vi "ElevatorSim_New.vi"(4 "Simulate Gravity":bool=TRUE, 5 "MaxHeight_Meters":dbl, 6 "DrumRadius_Meters":dbl, 7 "MinHeight_Meters":dbl, 8 "MeasurementStdDev":T1=[[0.0]], 9 "CarriageMass_Kg":dbl, 10 "Gearing":dbl=1.0, 11 "GearBox":T2 {"Jr_KgM2" format="%13.5p"; "L_H" format="%13.5p"; "Kt_NMPerAmp" format="%13.5p"; "KvINV_RadPerSecPerVolt" format="%13.5p"; "R_Ohms" format="%13.5p"; "FreeSpeed_RadPerSec" format="%13.5p"; "FreeCurrent_Amps" format="%13.5p"; "StallCurrent_Amps" format="%13.5p"; "StallTorque_NM" format="%13.5p"; "nominalVoltage_Volts" format="%13.5p"}) -> (0 "Error":bool, 3 "ElevatorSim":T3={"LinearSystemSim"={"m_Plant"={"m_A"=[], "m_B"=[], "m_C"=[], "m_D"=[], "States"=0, "Inputs"=0, "Outputs"=0}, "m_X"=[], "m_Y"=[], "m_U"=[], "MeasureStdDev"=[]}, "GearBox"={"nominalVoltage_Volts"=0.0, "StallTorque_NM"=0.0, "StallCurrent_Amps"=0.0, "FreeCurrent_Amps"=0.0, "FreeSpeed_RadPerSec"=0.0, "R_Ohms"=0.0, "KvINV_RadPerSecPerVolt"=0.0, "Kt_NMPerAmp"=0.0, "L_H"=0.0, "Jr_KgM2"=0.0}, "Gearing"=0.0, "DrumRadius_M"=0.0, "MinHeight_M"=0.0, "MaxHeight_M"=0.0, "CarriageMass_Kg"=0.0, "SimulateGravity"=TRUE} {"GearBox"."Jr_KgM2" format="%13.5p"; "GearBox"."L_H" format="%13.5p"; "GearBox"."Kt_NMPerAmp" format="%13.5p"; "GearBox"."KvINV_RadPerSecPerVolt" format="%13.5p"; "GearBox"."R_Ohms" format="%13.5p"; "GearBox"."FreeSpeed_RadPerSec" format="%13.5p"; "GearBox"."FreeCurrent_Amps" format="%13.5p"; "GearBox"."StallCurrent_Amps" format="%13.5p"; "GearBox"."StallTorque_NM" format="%13.5p"; "GearBox"."nominalVoltage_Volts" format="%13.5p"})   [LabVIEW 2019, in "Trajectory_Library.lvlib"]
doc: "Creates a simulated elevator mechanism.\n \nInputs:\n - maxHeightMeters -- The max allowable height of the elevator.\n - minHeightMeters -- The min allowable height of the elevator.\n - gearbox -- The type of and number of motors in the elevator gearbox.\n - gearing -- The gearing of the elevator (numbers greater than 1 represent reductions).\n - carriageMassKg -- The mass of the elevator carriage.\n - MeasurementStdDev -- Vector matrix of std deviations for measurements.\n - drumRadiusMeters -- The radius of the drum that the elevator spool is wrapped around.\n - SimulateGravity -- Simulate gravity (optional) Default: True\n\nOutputs:\n - OutElevatorSim -- Updated data cluster\n - Error -- If TRUE, an error occured."
uses:
  Trajectory_Library.lvlib
  <vilib>/Analysis/Matrix/Datatypes/RealMatrix.ctl
  <vilib>/Analysis/Matrix/NI_Matrix.lvlib
  TypeDef/LINEAR_SYSTEM.ctl
  TypeDef/DCMOTOR.CTL
  TypeDef/LINEAR_SYSTEM_SIM.ctl
  TypeDef/ELEVATOR_SIM.ctl
panel:
  # "<1, 1>"
  # "<States, 1>"
  # "<Outputs, 1>"
  # "<Inputs, 1>"
  # "<Outputs, 1>"
  # "<States,States>"
  # "<States,Inputs>"
  # "<Outputs,States>"
  # "<Outputs,Inputs>"
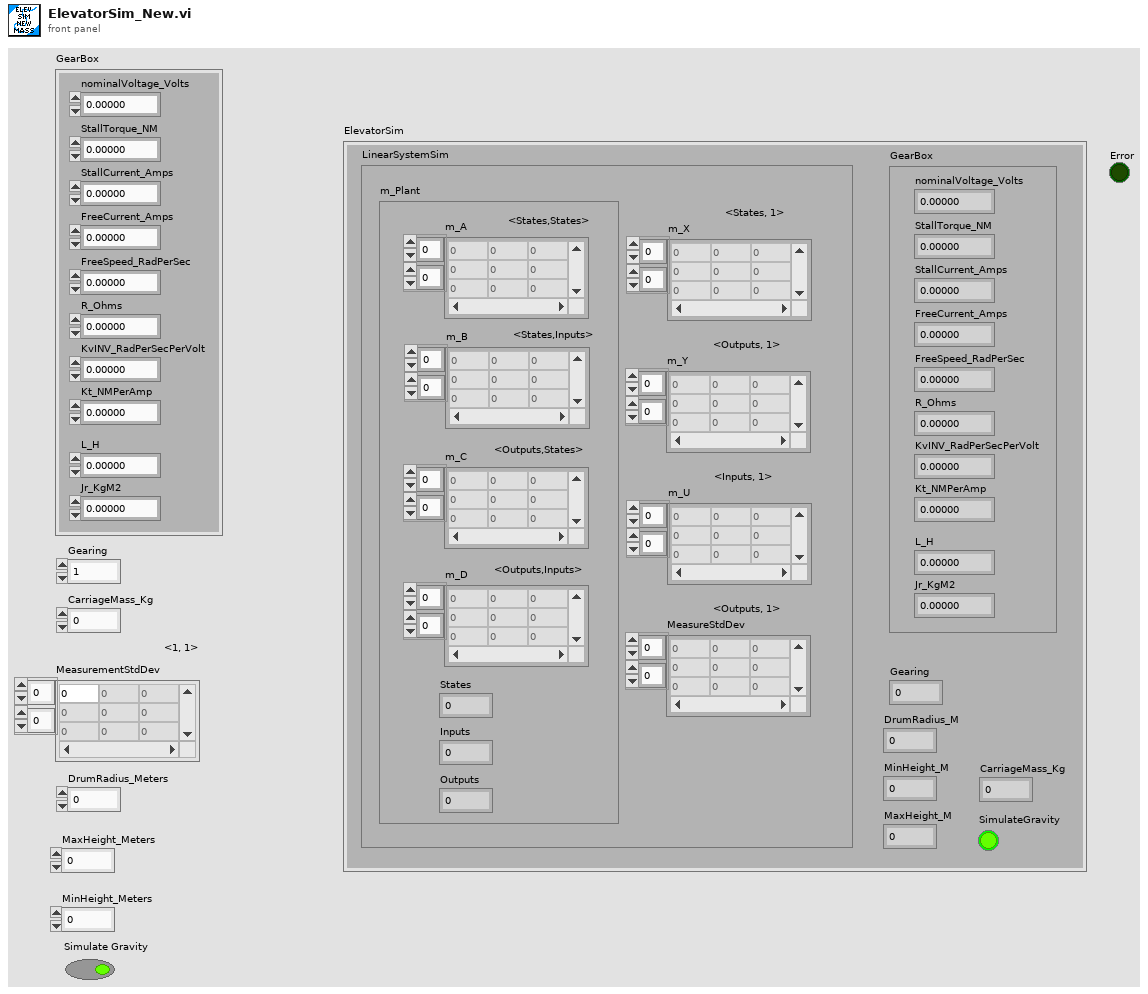
[diagram p1: front panel]
types:
  T1 = typedef "NI_Matrix.lvlib/RealMatrix.ctl" = dbl[][]
  T2 = typedef "Trajectory_Library.lvlib/DCMOTOR.CTL" = cluster{"nominalVoltage_Volts":dbl, "StallTorque_NM":dbl, "StallCurrent_Amps":dbl, "FreeCurrent_Amps":dbl, "FreeSpeed_RadPerSec":dbl, "R_Ohms":dbl, "KvINV_RadPerSecPerVolt":dbl, "Kt_NMPerAmp":dbl, "L_H":dbl, "Jr_KgM2":dbl}
  T3 = typedef "Trajectory_Library.lvlib/ELEVATOR_SIM.ctl" = cluster{"LinearSystemSim":T4, "GearBox":T2, "Gearing":dbl, "DrumRadius_M":dbl, "MinHeight_M":dbl, "MaxHeight_M":dbl, "CarriageMass_Kg":dbl, "SimulateGravity":bool}
  T4 = typedef "Trajectory_Library.lvlib/LINEAR_SYSTEM_SIM.ctl" = cluster{"m_Plant":T5, "m_X":T1, "m_Y":T1, "m_U":T1, "MeasureStdDev":T1}
  T5 = typedef "Trajectory_Library.lvlib/LINEAR_SYSTEM.ctl" = cluster{"m_A":T1, "m_B":T1, "m_C":T1, "m_D":T1, "States":i32, "Inputs":i32, "Outputs":i32}
  T6 = typedef "WPILib_Math.lvlib/LINEAR_SYSTEM.ctl" = cluster{"m_A":T1, "m_B":T1, "m_C":T1, "m_D":T1, "States":i32, "Inputs":i32, "Outputs":i32}
  T7 = typedef "WPILib_Math.lvlib/LINEAR_SYSTEM_SIM.ctl" = cluster{"m_Plant":T6, "m_X":T1, "m_Y":T1, "m_U":T1, "MeasureStdDev":T1}
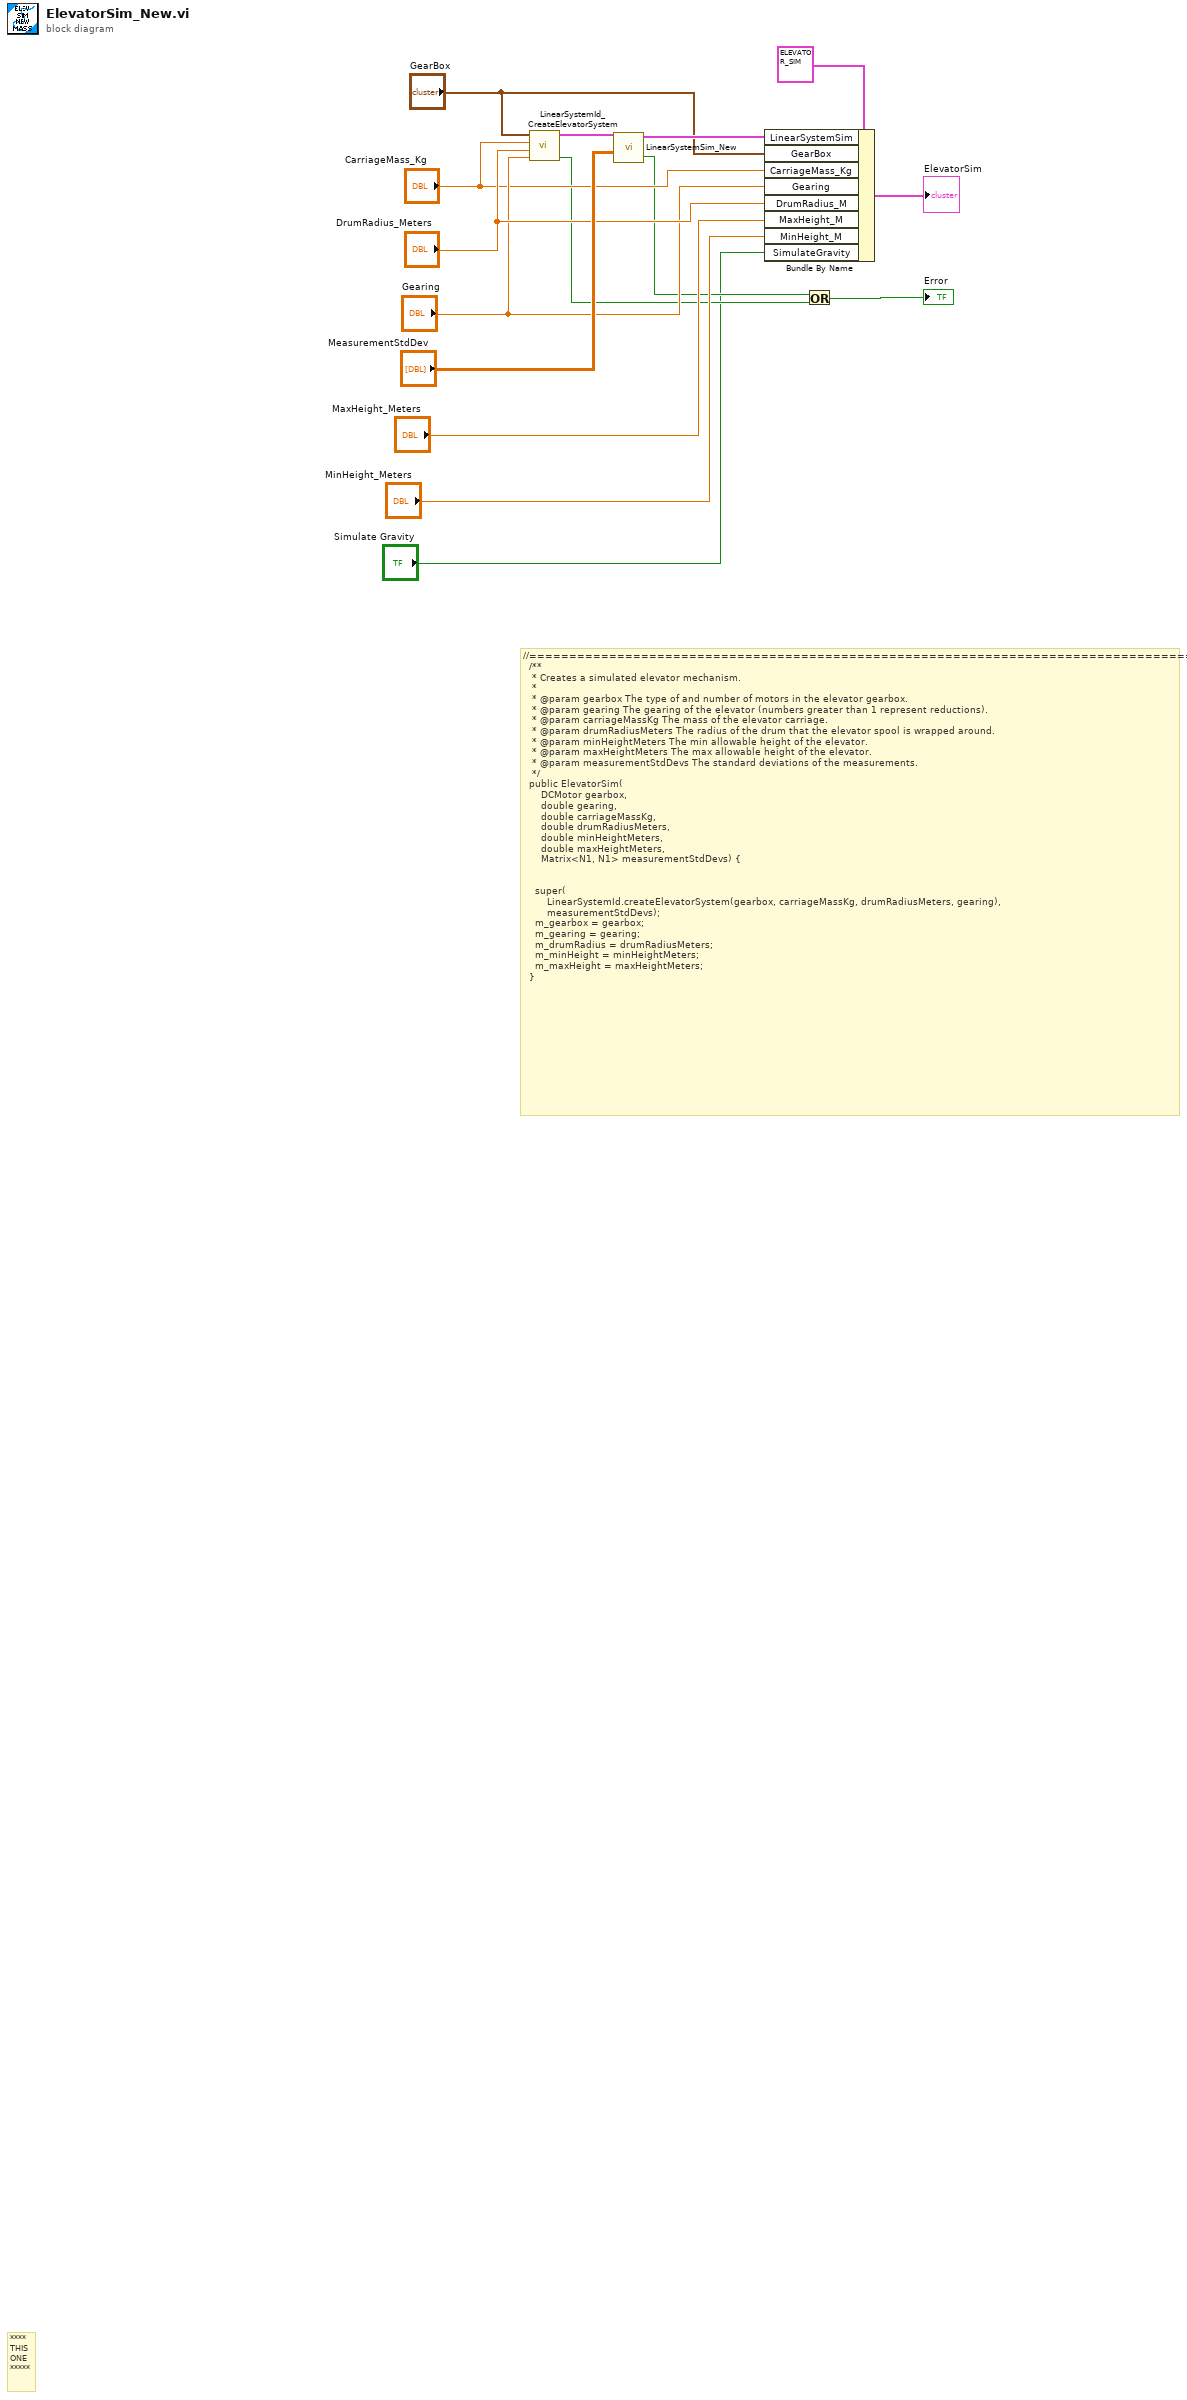
[diagram p0: block diagram]
diagram:
  # "//===================================================================================\n  /**\n   * Creates a simulated elevator mechanism.\n   *\n   * @param gearbox The type of and number of motors in the elevator gearbox.\n   * @param gearing The gearing of the elevator (numbers greater than 1 represent reductions).\n   * @param carriageMassKg The mass of the elevator carriage.\n   * @param drumRadiusMeters The radius of the drum that the elevator spool is wrapped around.\n   * @param minHeightMeters The min allowable height of the elevator.\n   * @param maxHeightMeters The max allowable height of the elevator.\n   * @param measurementStdDevs The standard deviations of the measurements.\n   */\n  public ElevatorSim(\n      DCMotor gearbox,\n      double gearing,\n      double carriageMassKg,\n      double drumRadiusMeters,\n      double minHeightMeters,\n      double maxHeightMeters,\n      Matrix<N1, N1> measurementStdDevs) {\n\n\n    super(\n        LinearSystemId.createElevatorSystem(gearbox, carriageMassKg, drumRadiusMeters, gearing),\n        measurementStdDevs);\n    m_gearbox = gearbox;\n    m_gearing = gearing;\n    m_drumRadius = drumRadiusMeters;\n    m_minHeight = minHeightMeters;\n    m_maxHeight = maxHeightMeters;\n  }"
  # "****\nTHIS\nONE\n*****"
  n1 = call "LinearSystemId_CreateElevatorSystem.vi"("G"="Gearing", "radiusMeters"="DrumRadius_Meters", "massKg"="CarriageMass_Kg", "DCMOTOR"="GearBox") -> ("Size Coerced"=w3:bool, "Linearsystem"=w11:T6)  [unwired: 6 in]
  n2 = call "LinearSystemSim_New.vi"("MeasurementStdDev"="MeasurementStdDev", "System"=w11) -> ("Size Coerced"=w4:bool, "LinearSystemSim"=w13:T7)  [unwired: 8 in]
  n3 = Bundle By Name(cluster=T3 {"LinearSystemSim"={"m_Plant"={"m_A"=[], "m_B"=[], "m_C"=[], "m_D"=[], "States"=0, "Inputs"=0, "Outputs"=0}, "m_X"=[], "m_Y"=[], "m_U"=[], "MeasureStdDev"=[]}, "GearBox"={"nominalVoltage_Volts"=0.0, "StallTorque_NM"=0.0, "StallCurrent_Amps"=0.0, "FreeCurrent_Amps"=0.0, "FreeSpeed_RadPerSec"=0.0, "R_Ohms"=0.0, "KvINV_RadPerSecPerVolt"=0.0, "Kt_NMPerAmp"=0.0, "L_H"=0.0, "Jr_KgM2"=0.0}, "Gearing"=0.0, "DrumRadius_M"=0.0, "MinHeight_M"=0.0, "MaxHeight_M"=0.0, "CarriageMass_Kg"=0.0, "SimulateGravity"=TRUE} ("ELEVATOR_SIM"), "LinearSystemSim"=w13, "GearBox"="GearBox", "CarriageMass_Kg"="CarriageMass_Kg", "Gearing"="Gearing", "DrumRadius_M"="DrumRadius_Meters", "MaxHeight_M"="MaxHeight_Meters", "MinHeight_M"="MinHeight_Meters", "SimulateGravity"="Simulate Gravity") -> (→"ElevatorSim":T3)
  n4 = Or(x=w4, y=w3) -> (x .or. y?=→"Error":bool)
